vi "APS motion status.vi"(8 "error in (no error)":errorcluster caption="错误输入（无错误）", 11 "Axis_ID":i32) -> (0 "error out":errorcluster caption="错误输出", 1 "x与y?":bool)   [LabVIEW 2017, in "APS168.lvlib"]
doc: "I32 FNTYPE APS_motion_status( I32 Axis_ID );"
uses:
  APS168.lvlib
  APS168.dll
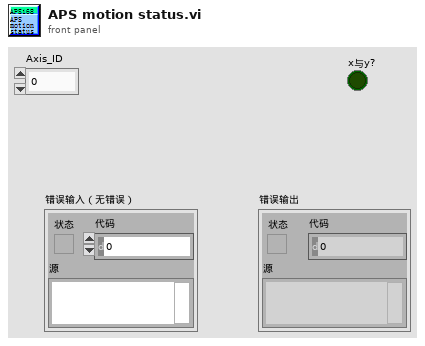
[diagram p1: front panel]
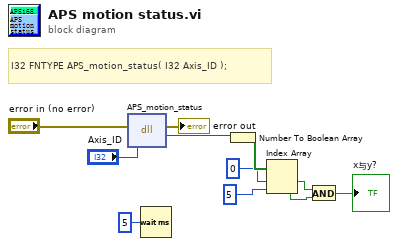
[diagram p0: block diagram]
diagram:
  # "I32 FNTYPE APS_motion_status( I32 Axis_ID );"
  n1 = dll-call lib="PTH2Labs E迈治LV范例testSubVIsADLINKLLB运动204cAPS168.*" fn="APS_motion_status"(error in="error in (no error)", "Axis_ID"="Axis_ID") -> (error out=→"error out":errorcluster, "return type"=w2:i32)  [unwired: 3 in, 1 out]
  n2 = Wait (ms)(milliseconds to wait=u32 5 ("等待时间（毫秒）")) -> ()  [unwired: 1 out]
  n3 = Number To Boolean Array(number=w2) -> (Boolean array=w7:bool[])
  n4 = Index Array(array=w7, index #1=0 ("索引"), index #2=5 ("索引")) -> (element #1=w4:bool, element #2=w3:bool)
  n5 = And(x=w4, y=w3) -> (x .and. y?=→"x与y?":bool)
